vi "NeutralZone.vi"(8 "error in":errorcluster, 10 "Alliance":enum16{"Blue", "Red"}(ring), 11 "Gear Side":enum16{"Center", "Left", "Right"}(ring)) -> (0 "error out":errorcluster)   [LabVIEW 2016]
doc: "Robot drives into neutral zone to save time and other strategic advanteges"
uses:
  Robot Global Data.vi
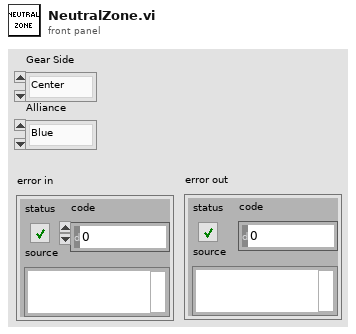
[diagram p1: front panel]
types:
  T1 = cluster{"InchesBack":dbl, "Degrees":dbl, "InchesBack2":dbl, "Degrees2":dbl, "InchesBack3":dbl}
  T2 = cluster{"InchesBack":dbl, "Degrees":dbl, "InchesBack2":dbl, "Degrees2":dbl, "InchesBack3":dbl, "Degrees3":dbl}
  T3 = cluster{"InchesBack":dbl, "Degrees":dbl, "InchesBack2":dbl}
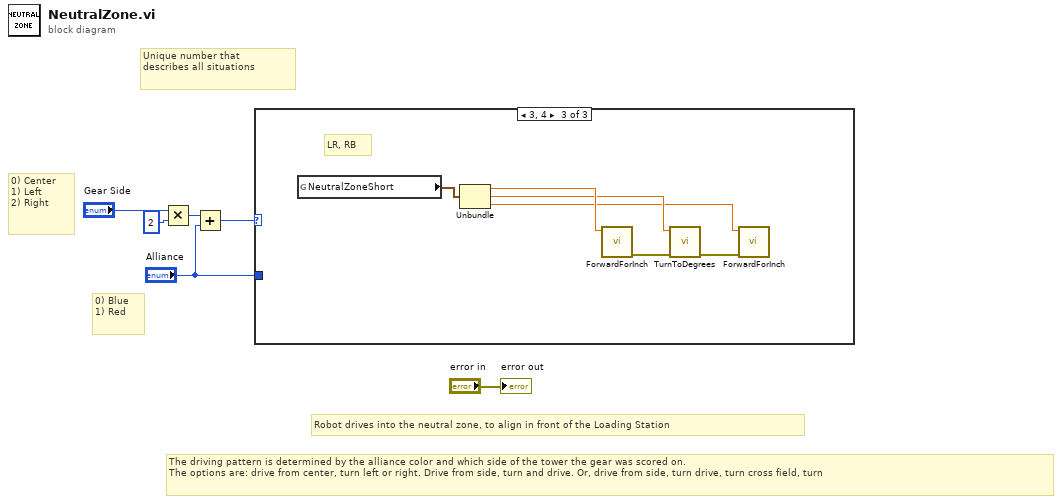
[diagram p0: block diagram]
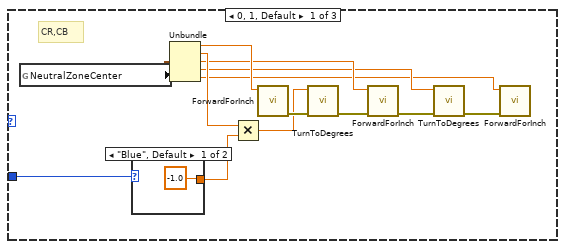
[diagram p2: hidden frame]
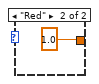
[diagram p3: hidden frame]
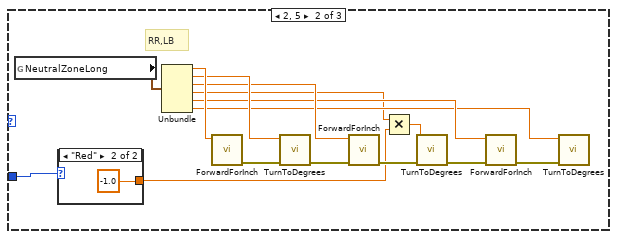
[diagram p4: hidden frame]
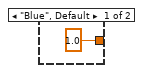
[diagram p5: hidden frame]
diagram:
  # "Unique number that\ndescribes all situations"
  # "0) Blue\n1) Red"
  # "0) Center\n1) Left\n2) Right"
  # "The driving pattern is determined by the alliance color and which side of the tower the gear was scored on.\nThe options are: drive from center, turn left or right. Drive from side, turn and drive. Or, drive from side, turn drive, turn cross field, turn"
  # "Robot drives into the neutral zone, to align in front of the Loading Station"
  n1 = Multiply(x="Gear Side", y=2) -> (x*y=w3:i32)
  n2 = Add(x=w3, y="Alliance") -> (x+y=w2:i32)
  n3 = case shown="3, 4" w2 {
    tunnel: "Alliance" -> [w19 w26 _]
    frame 0, 1, Default {
      # "CR,CB"
      n4 = global read "Robot Global Data.vi" "NeutralZoneCenter"() -> (w14:T1)
      n5 = case shown="\"Blue\", Default" w19 {
        tunnel: [-1.0 ("Distance") 1.0 ("Distance")] -> w11
        frame "Blue", Default {
        }
        frame "Red" {
        }
      }
      n6 = Unbundle(w14) -> ("InchesBack"=w13:dbl, "Degrees"=w12:dbl, "InchesBack2"=w9:dbl, "Degrees2"=w8:dbl, "InchesBack3"=w7:dbl)
      n7 = Multiply(x=w12, y=w11) -> (x*y=w10:dbl)
      n8 = call "ForwardForInch.vi"("Distance"=w13) -> ("error out"=w18:errorcluster)  [unwired: 10 in]
      n9 = call "TurnToDegrees.vi"("error in"=w18, "Angle"=w10) -> ("error out"=w16:errorcluster)  [unwired: 9 in]
      n10 = call "ForwardForInch.vi"("error in"=w16, "Distance"=w9) -> ("error out"=w17:errorcluster)  [unwired: 9 in]
      n11 = call "TurnToDegrees.vi"("error in"=w17, "Angle"=w8) -> ("error out"=w15:errorcluster)  [unwired: 9 in]
      n12 = call "ForwardForInch.vi"("error in"=w15, "Distance"=w7) -> ()  [unwired: 9 in, 1 out]
    }
    frame 2, 5 {
      # "RR,LB"
      n13 = global read "Robot Global Data.vi" "NeutralZoneLong"() -> (w22:T2)
      n14 = case shown="\"Red\"" w26 {
        tunnel: [1.0 -1.0] -> w24
        frame "Blue", Default {
        }
        frame "Red" {
        }
      }
      n15 = Unbundle(w22) -> ("InchesBack"=w31:dbl, "Degrees"=w30:dbl, "InchesBack2"=w29:dbl, "Degrees2"=w23:dbl, "InchesBack3"=w28:dbl, "Degrees3"=w27:dbl)
      n16 = call "ForwardForInch.vi"("Distance"=w31) -> ("error out"=w36:errorcluster)  [unwired: 10 in]
      n17 = call "TurnToDegrees.vi"("error in"=w36, "Angle"=w30) -> ("error out"=w34:errorcluster)  [unwired: 9 in]
      n18 = call "ForwardForInch.vi"("error in"=w34, "Distance"=w29) -> ("error out"=w35:errorcluster)  [unwired: 9 in]
      n19 = Multiply(x=w23, y=w24) -> (x*y=w25:dbl)
      n20 = call "TurnToDegrees.vi"("error in"=w35, "Angle"=w25) -> ("error out"=w33:errorcluster)  [unwired: 9 in]
      n21 = call "ForwardForInch.vi"("error in"=w33, "Distance"=w28) -> ("error out"=w32:errorcluster)  [unwired: 9 in]
      n22 = call "TurnToDegrees.vi"("error in"=w32, "Angle"=w27) -> ()  [unwired: 9 in, 1 out]
    }
    frame 3, 4 {
      # "LR, RB"
      n23 = global read "Robot Global Data.vi" "NeutralZoneShort"() -> (w42:T3)
      n24 = Unbundle(w42) -> ("InchesBack"=w41:dbl, "Degrees"=w40:dbl, "InchesBack2"=w39:dbl)
      n25 = call "ForwardForInch.vi"("Distance"=w41) -> ("error out"=w44:errorcluster)  [unwired: 10 in]
      n26 = call "TurnToDegrees.vi"("error in"=w44, "Angle"=w40) -> ("error out"=w43:errorcluster)  [unwired: 9 in]
      n27 = call "ForwardForInch.vi"("error in"=w43, "Distance"=w39) -> ()  [unwired: 9 in, 1 out]
    }
  }
  "error out" <- "error in"
